vi "SI8_Query.vi"(7 "String":string, 8 "error in (no error)":errorcluster, 11 "DriverConnect in":T1) -> (0 "error out":errorcluster, 3 "DriverConnect out":T1, 4 "String from device out":string)   [LabVIEW 2018]
uses:
  MOKO_LabViewLibrary/MokoLowLevel/MokoLowLovelControl/MLLC_ConnectCluster.ctl
  MOKO_LabViewLibrary/MokoLowLevel/MokoLowLovelControl/MLLC_InterfaceType.ctl
  MOKO_LabViewLibrary/MokoLowLevel/MokoLowLovelControl/MLLC_OpenedSession.ctl
  MOKO_LabViewLibrary/MokoLowLevel/MokoLowLovelControl/MLLC_InterfaceSettings.ctl
  MOKO_LabViewLibrary/MokoLowLevel/MokoLowLovelControl/MLLC_InterfaceKind.ctl
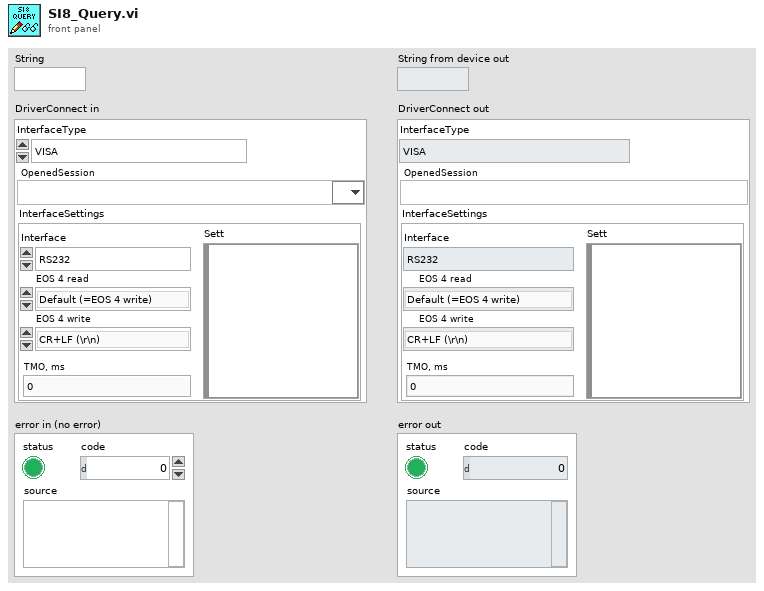
[diagram p1: front panel]
types:
  T1 = typedef "MLLC_ConnectCluster.ctl" = cluster{"InterfaceType":T2, "OpenedSession":T3, "InterfaceSettings":T4}
  T2 = typedef "MLLC_InterfaceType.ctl" = enum16{"VISA", "Prologix USB-GPIB"}
  T3 = typedef "MLLC_OpenedSession.ctl" = refnum<visa-resource-name>
  T4 = typedef "MLLC_InterfaceSettings.ctl" = cluster{"Interface":T5, "EOS 4 read":enum16{"Default (=EOS 4 write)", "CR (\\r)", "LF (\\n)", "None"}, "EOS 4 write":enum16{"CR+LF (\\r\\n)", "CR (\\r)", "LF (\\n)", "None"}, "TMO, ms":i32, "Sett":variant}
  T5 = typedef "MLLC_InterfaceKind.ctl" = enum16{"RS232", "GPIB", "USB", "Ethernet", "another"}
  T6 = typedef "MLLC_Error.ctl" = errorcluster
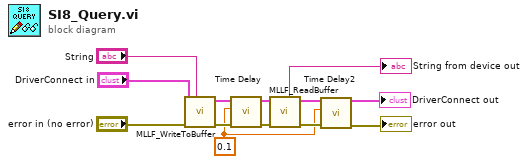
[diagram p0: block diagram]
diagram:
  w2 = 0.1 ("Delay Time (s)")
  n1 = call "MLLF_WriteToBuffer.vi"("String"="String", "error in"="error in (no error)", "DriverConnect in"="DriverConnect in") -> ("error out"=w8:T6, "DriverConnect out"=w6:T1)  [unwired: 5 in]
  n2 = call "Time Delay"("error in (no error)"=w8, "Delay Time (s)"=w2) -> ("error out"=w9:errorcluster)  [unwired: 9 in]
  n3 = call "MLLF_ReadBuffer.vi"("Error In"=w9, "DriverConnect in"=w6) -> ("Error Out"=w3:errorcluster, "DriverConnect out"=→"DriverConnect out":T1, "String"=→"String from device out":string)  [unwired: 6 in]
  n4 = call "Time Delay2"("error in (no error)"=w3, "Delay Time (s)"=w2) -> ("error out"=→"error out":errorcluster)  [unwired: 9 in]
